vi "Sim_Eminem.vi"(9 "Motor Dmd C":dbl, 10 "Motor Dmd B":dbl, 11 "Motor Dmd A":dbl) -> (1 "MotorRPM C":dbl, 2 "MotorRPM B":dbl, 3 "MotorRPM A":dbl)   [LabVIEW 2023]
uses:
  <vilib>/Rock Robotics/WPI/ThirdParty/JAS_Junk/TrajLib/Enum/DCMOTOR_TYPES_ENUM.ctl
  <vilib>/Rock Robotics/WPI/ThirdParty/JAS_Junk/TrajLib/BatterySim_CalculateLoadedBatteryVoltage.vi
  <vilib>/Rock Robotics/WPI/ThirdParty/JAS_Junk/TrajLib/Trajectory_Library.lvlib
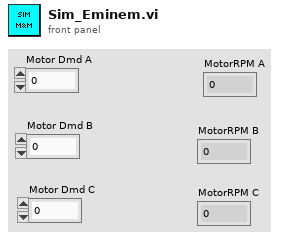
[diagram p1: front panel]
types:
  T1 = typedef "Trajectory_Library.lvlib/DCMOTOR_TYPES_ENUM.ctl" = enum16{"CIM", "AndyMark 9015", "Andy Mark RS 775 125", "Bag", "BaneBots RS 550", "BaneBots RS 775", "Falcon 500", "Mini CIM", "NEO", "NEO 550", "Romi BuiltIn", "Vex 775 Pro", "Snow Blower AM 2235A", "Bosch Seat AM 3493"}
  T2 = typedef "Trajectory_Library.lvlib/LINEAR_SYSTEM_ID_FLYWHEEL_MODEL.ctl" = cluster{"DCMOTOR_TYPES":T1, "Num Motors":i32, "Gearing":dbl, "MOI kgm2":dbl}
  T3 = typedef "Trajectory_Library.lvlib/FLYWHEEL_SIM_SIMULATION_PARAMS.ctl" = cluster{"Vel Meas Std Dev Rad/Sec":dbl}
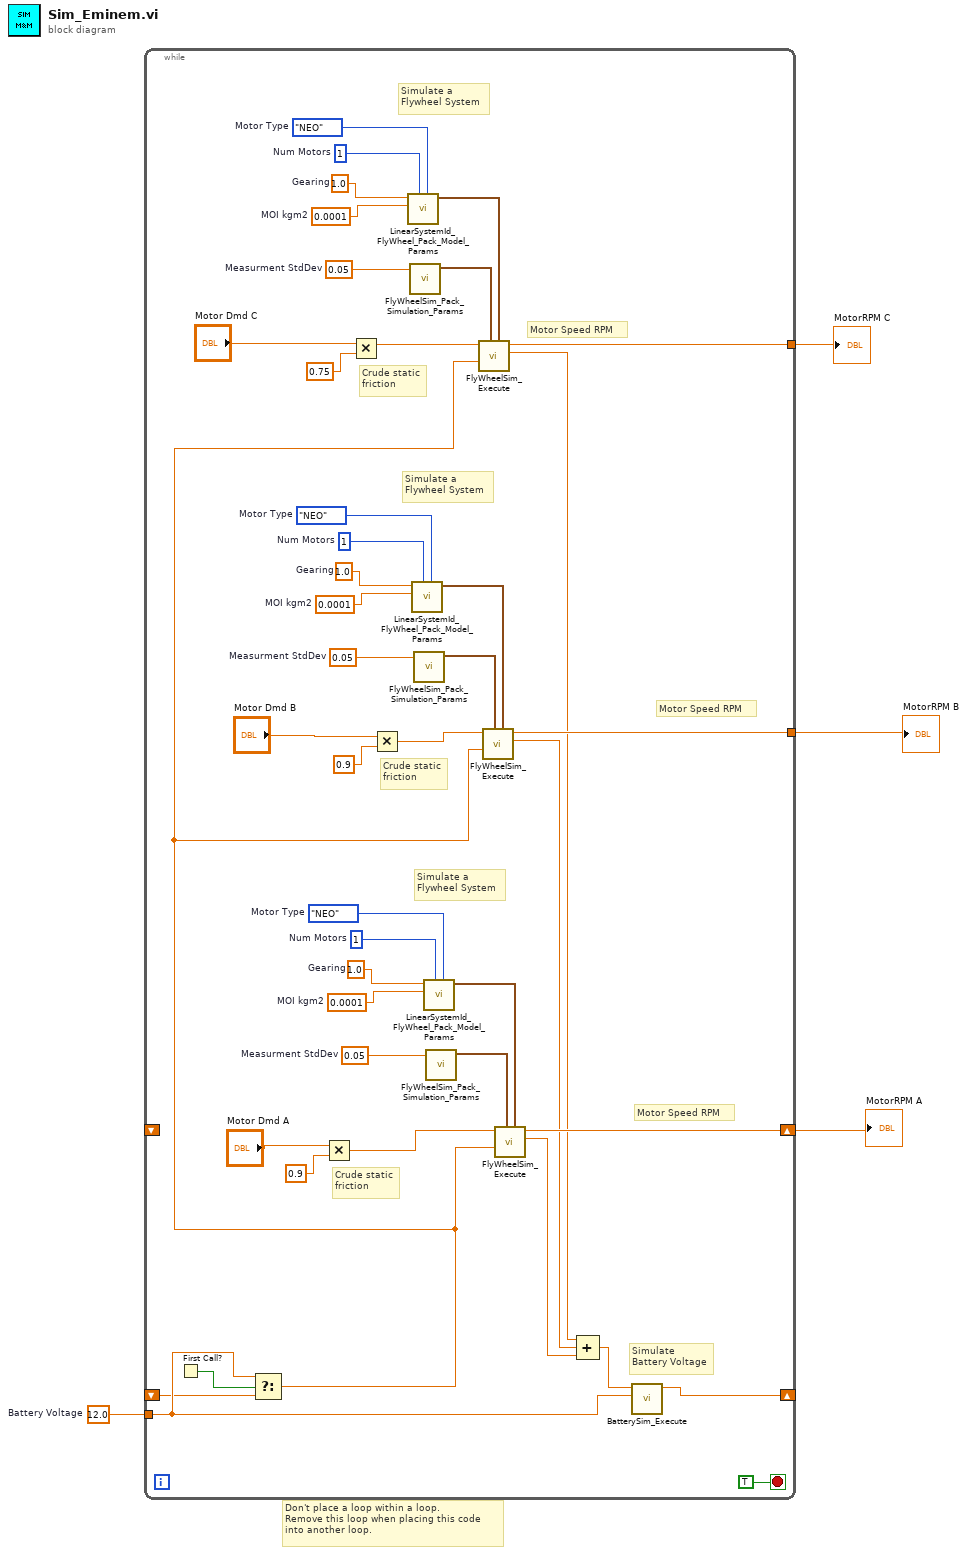
[diagram p0: block diagram]
diagram:
  w4 = 12.0  # Battery Voltage
  # "Don't place a loop within a loop. \nRemove this loop when placing this code\ninto another loop."
  n1 = while {
    shift-right: [w46] -> _
    shift-left: _ -> [w41]
    shift-right: [w19] -> w1
    shift-left: _ -> [_]
    tunnel: w4 -> [w42]
    tunnel: [w15] -> w2
    tunnel: [w14] -> w3
    stop <- TRUE stop-if-true
    w24 = 0.05  # Measurment StdDev
    w20 = 1.0  # Gearing
    w21 = 0.0001  # MOI kgm2
    w22 = 1  # Num Motors
    w23 = DCMOTOR_TYPES_ENUM."NEO"  # Motor Type
    w31 = 0.05  # Measurment StdDev
    w27 = 1.0  # Gearing
    w28 = 0.0001  # MOI kgm2
    w29 = 1  # Num Motors
    w30 = DCMOTOR_TYPES_ENUM."NEO"  # Motor Type
    w38 = 0.05  # Measurment StdDev
    w34 = 1.0  # Gearing
    w35 = 0.0001  # MOI kgm2
    w36 = 1  # Num Motors
    w37 = DCMOTOR_TYPES_ENUM."NEO"  # Motor Type
    # "Crude static\nfriction"
    # "Crude static\nfriction"
    # "Motor Speed RPM"
    # "Simulate a \nFlywheel System"
    # "Motor Speed RPM"
    # "Simulate a \nFlywheel System"
    # "Motor Speed RPM"
    # "Simulate a \nFlywheel System"
    # "Crude static\nfriction"
    # "Simulate\nBattery Voltage"
    n2 = First Call?() -> (First Call?: T/F=w43:bool)
    n3 = Select(t=w42, s=w43, f=w41) -> (s? t:f=w10:dbl)
    n4 = Multiply(x="Motor Dmd A", y=0.9) -> (x*y=w16:dbl)
    n5 = Multiply(x="Motor Dmd C", y=0.75) -> (x*y=w6:dbl)
    n6 = Multiply(x="Motor Dmd B", y=0.9) -> (x*y=w8:dbl)
    n7 = call <vilib>:"LinearSystemId_FlyWheel_Pack_Model_Params.vi"("DCMOTOR_TYPES"=w37, "Num Motors"=w36, "MOI kgm2"=w35, "Gearing"=w34) -> ("LinearSystem_ID_FlyWheel_Model"=w39:T2)  [unwired: 7 in]
    n8 = call <vilib>:"FlyWheelSim_Pack_Simulation_Params.vi"("Vel Meas StdDev Rad/Sec"=w38) -> ("FlyWheelSim_Simulation_Params"=w40:T3)  [unwired: 10 in]
    n9 = call <vilib>:"LinearSystemId_FlyWheel_Pack_Model_Params.vi"("DCMOTOR_TYPES"=w30, "Num Motors"=w29, "MOI kgm2"=w28, "Gearing"=w27) -> ("LinearSystem_ID_FlyWheel_Model"=w32:T2)  [unwired: 7 in]
    n10 = call <vilib>:"FlyWheelSim_Pack_Simulation_Params.vi"("Vel Meas StdDev Rad/Sec"=w31) -> ("FlyWheelSim_Simulation_Params"=w33:T3)  [unwired: 10 in]
    n11 = call <vilib>:"LinearSystemId_FlyWheel_Pack_Model_Params.vi"("DCMOTOR_TYPES"=w23, "Num Motors"=w22, "MOI kgm2"=w21, "Gearing"=w20) -> ("LinearSystem_ID_FlyWheel_Model"=w25:T2)  [unwired: 7 in]
    n12 = call <vilib>:"FlyWheelSim_Pack_Simulation_Params.vi"("Vel Meas StdDev Rad/Sec"=w24) -> ("FlyWheelSim_Simulation_Params"=w26:T3)  [unwired: 10 in]
    n13 = call <vilib>:"FlyWheelSim_Execute.vi"("FlyWheelSim_Model _Params"=w39, "FlyWheelSim_Simulation_Params"=w40, "Battery Volts"=w10, "Motor Dmd"=w6) -> ("Motor Current"=w12:dbl, "Velocity_RPM"=w14:dbl)  [unwired: 4 in, 2 out]
    n14 = call <vilib>:"FlyWheelSim_Execute.vi"("FlyWheelSim_Model _Params"=w32, "FlyWheelSim_Simulation_Params"=w33, "Battery Volts"=w10, "Motor Dmd"=w8) -> ("Motor Current"=w13:dbl, "Velocity_RPM"=w15:dbl)  [unwired: 4 in, 2 out]
    n15 = call <vilib>:"FlyWheelSim_Execute.vi"("FlyWheelSim_Model _Params"=w25, "FlyWheelSim_Simulation_Params"=w26, "Battery Volts"=w10, "Motor Dmd"=w16) -> ("Motor Current"=w17:dbl, "Velocity_RPM"=w19:dbl)  [unwired: 4 in, 2 out]
    n16 = Compound Arithmetic op=ADD(w12, w13, w17) -> (w18:dbl)
    n17 = call <vilib>:"BatterySim_Execute.vi"("Nominal Battery Voltage"=w42, "Current"=w18) -> ("Voltage"=w46:dbl)  [unwired: 9 in]
  }
  "MotorRPM A" <- w1
  "MotorRPM B" <- w2
  "MotorRPM C" <- w3
